vi "Merge.vi"(8 "error in (no error)":errorcluster, 9 "Target":string, 10 "Git Implementation":refnum<class "Git Implementation.lvclass">, 11 "Git-Merger in":refnum<class "Merge-Delegate.lvclass">) -> (0 "error out":errorcluster, 2 "Status Message":string)   [LabVIEW 2017, in "Git-LabVIEW.lvlib" / "Merge-Delegate.lvclass"]
doc: "Perform a merge of the \"Target\" into the current branch. If Target is not specified, then the branch will merge \"the remote-tracking branches that the current branch is configured to use as its upstream\".\nSee https://git-scm.com/docs/git-merge for more details.\nThe Status Message is for display only, and cannot be guaranteed for use with scripting."
uses:
  Merge-Delegate.lvclass
  Implementation/Git Implementation.lvclass
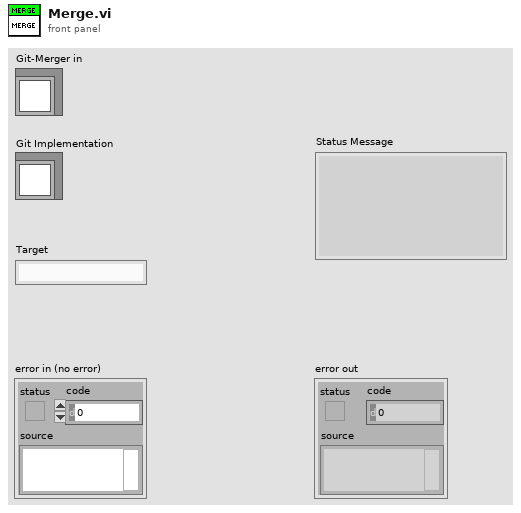
[diagram p1: front panel]
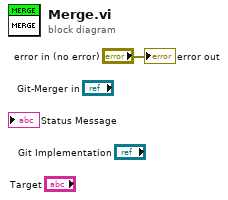
[diagram p0: block diagram]
diagram:
  "error out" <- "error in (no error)"
